vi "bk9132b Read_Chxx.vi"(7 "Chanel (1-3)":u8, 11 "VISA resource name":refnum<visa-resource-name>) -> (0 "error out":errorcluster, 1 "Actual Power":dbl format="%.4g", 2 "Actual Current":dbl format="%.4g", 3 "Actual Voltage":dbl format="%.4g")   [LabVIEW 2018]
uses:
  <instrlib>/BK Precision 913XX/BK Precision 913XX.lvlib
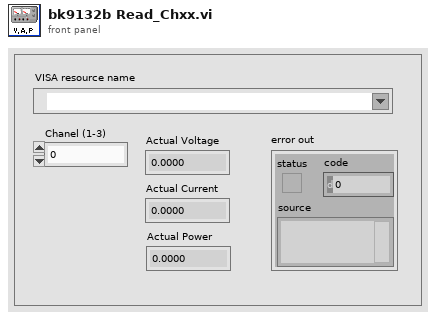
[diagram p1: front panel]
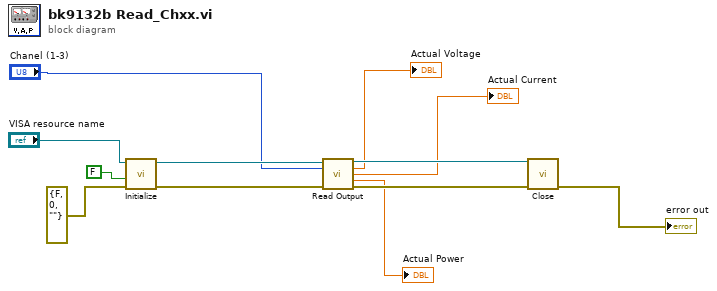
[diagram p0: block diagram]
diagram:
  n1 = call <instrlib>:"Initialize.vi"("error in (no error)"=errorcluster {"status"=FALSE, "code"=0, "source"=""}, "Reset (True)"=FALSE, "VISA resource name"="VISA resource name") -> ("error out"=w8:errorcluster, "VISA resource name out"=w6:refnum<visa-resource-name>)  [unwired: 7 in]
  n2 = call <instrlib>:"Read Output.vi"("VISA resource name"=w6, "Channel (1:Channel 1)"="Chanel (1-3)", "error in (no error)"=w8) -> ("VISA resource name out"=w5:refnum<visa-resource-name>, "Actual Voltage Level (V)"=→"Actual Voltage":dbl, "Actual Current Level (A)"=→"Actual Current":dbl, "Actual Power Level (W)"=→"Actual Power":dbl, "error out"=w7:errorcluster)  [unwired: 8 in]
  n3 = call <instrlib>:"Close.vi"("error in (no error)"=w7, "VISA resource name"=w5) -> ("error out"=→"error out":errorcluster)  [unwired: 9 in]
